vi "Email_transfer_global.vi"() -> ()   [LabVIEW 2010]
panel:
  in  "Started sending":timestamp
  in  "Busy?":bool
  in  "attachments":T1(array[cluster])
  in  "message":string
  in  "subject ([No Subject])":string="[No Subject]"
  in  "recipients":string[](array[string])
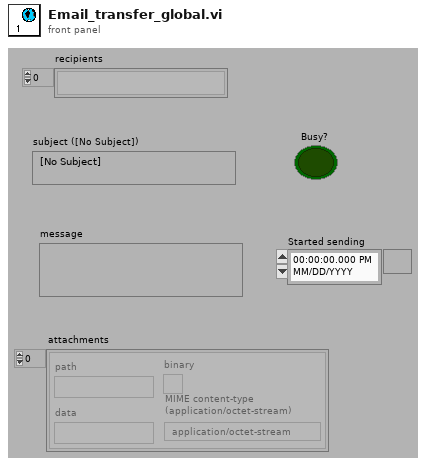
[diagram p1: front panel]
types:
  T1 = cluster{"path":path, "data":string, "binary":bool, "MIME content-type \n(application/octet-stream)":string}[]
diagram:
